vi "Select Limit Line Actions.vi"(0 "VISA resource name":refnum<visa-resource-name>, 5 "Limit Line Settings (0:Create)":u16(ring) items=["Create", "Update", "Delete", "Delete All"], 7 "Limit Line (1)":i32=1 min=1 max=6, 11 "error in (no error)":errorcluster) -> (4 "VISA resource name out":refnum<visa-resource-name>, 15 "error out":errorcluster)   [LabVIEW 2020, in "Anritsu Signal Analyzer Series.lvlib"]
doc: "Creates, Updates, or Deletes (single or all) Limit Points of the currently selected Limit."
uses:
  Anritsu Signal Analyzer Series.lvlib
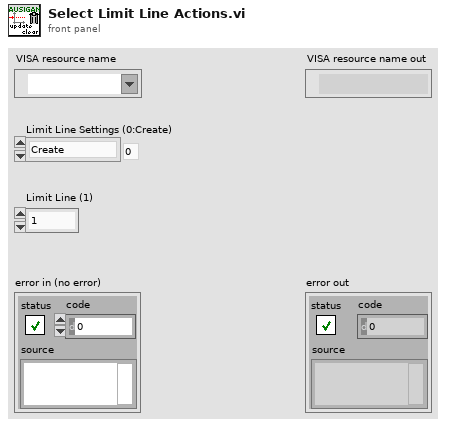
[diagram p1: front panel]
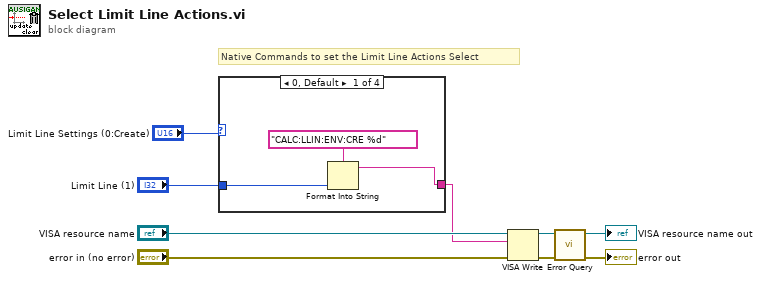
[diagram p0: block diagram]
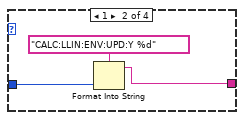
[diagram p2: hidden frame]
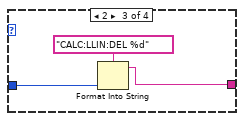
[diagram p3: hidden frame]
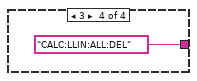
[diagram p4: hidden frame]
diagram:
  # "Native Commands to set the Limit Line Actions Select"
  n1 = case shown="0, Default" "Limit Line Settings (0:Create)" {
    tunnel: [w11 w14 w17 "CALC:LLIN:ALL:DEL" ("_Command")] -> w5
    tunnel: "Limit Line (1)" -> [w10 w13 w16 _]
    frame 0, Default {
      n2 = Format Into String(format string="CALC:LLIN:ENV:CRE %d" ("_Command"), w10) -> (resulting string=w11:string)  [unwired: 2 in, 1 out]
    }
    frame 1 {
      n3 = Format Into String(format string="CALC:LLIN:ENV:UPD:Y %d" ("_Command"), w13) -> (resulting string=w14:string)  [unwired: 2 in, 1 out]
    }
    frame 2 {
      n4 = Format Into String(format string="CALC:LLIN:DEL %d" ("_Command"), w16) -> (resulting string=w17:string)  [unwired: 2 in, 1 out]
    }
    frame 3 {
    }
  }
  n5 = VISA Write(VISA resource name="VISA resource name", write buffer=w5, error in (no error)="error in (no error)") -> (VISA resource name out=w3:refnum<visa-resource-name>, error out=w4:errorcluster)  [unwired: 1 out]
  n6 = call "Error Query.vi"("error in (no error)"=w4, "VISA resource name"=w3) -> ("error out"=→"error out":errorcluster, "VISA resource name out"=→"VISA resource name out":refnum<visa-resource-name>)  [unwired: 6 in, 2 out]
